vi "Get Channels limits.vi"(8 "error in (no error)":errorcluster, 9 "Power Supply In Use":T1, 10 "External Supply?":bool=TRUE, 11 "Channels":u16[](array[numeric])) -> (0 "error out":errorcluster, 3 "output cluster":T2)   [LabVIEW 2018, in "NI PXI-4110 Programmable Power Supply Custom Device.lvlib"]
uses:
  NI PXI-4110 Programmable Power Supply Custom Device.lvlib
  Power_Supply_In_Use.ctl
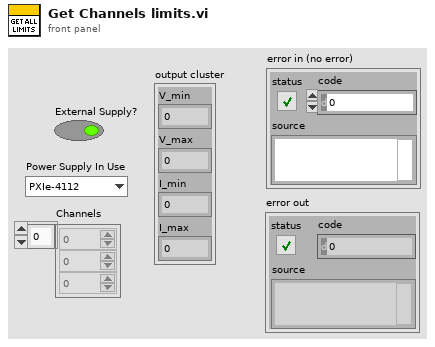
[diagram p1: front panel]
types:
  T1 = typedef "NI PXI-4110 Programmable Power Supply Custom Device.lvlib/Power_Supply_In_Use.ctl" = enum16{"PXIe-4112", "PXI-4110"}
  T2 = cluster{"V_min":dbl, "V_max":dbl, "I_min":dbl, "I_max":dbl}
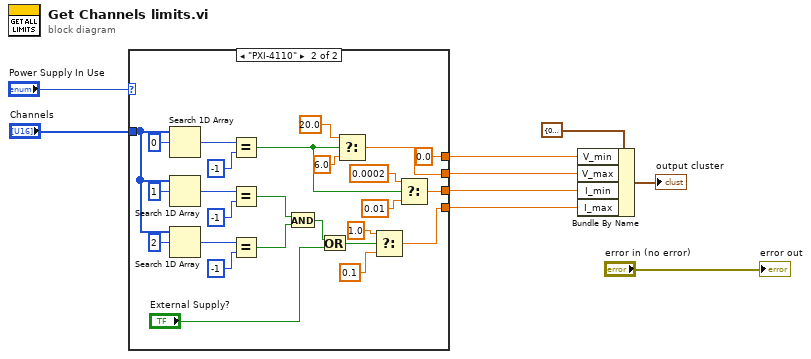
[diagram p0: block diagram]
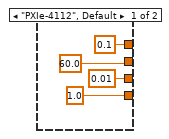
[diagram p2: hidden frame]
diagram:
  n1 = case shown="\"PXI-4110\"" "Power Supply In Use" {
    tunnel: [1.0 ("V_min") w21] -> w8
    tunnel: [0.01 ("V_min") w24] -> w7
    tunnel: [60.0 ("V_min") w26] -> w6
    tunnel: [0.1 ("V_min") 0.0 ("V_min")] -> w5
    tunnel: "Channels" -> [_ w30]
    frame "PXIe-4112", Default {
    }
    frame "PXI-4110" {
      n2 = Search 1D Array(1D array=w30, element=u16 0) -> (index of element=w38:i32)  [unwired: 1 in]
      n3 = Search 1D Array(1D array=w30, element=u16 1) -> (index of element=w35:i32)  [unwired: 1 in]
      n4 = Search 1D Array(1D array=w30, element=u16 2) -> (index of element=w32:i32)  [unwired: 1 in]
      n5 = Equal?(x=w38, y=-1) -> (x = y?=w25:bool)
      n6 = Equal?(x=w35, y=-1) -> (x = y?=w20:bool)
      n7 = Equal?(x=w32, y=-1) -> (x = y?=w19:bool)
      n8 = And(x=w20, y=w19) -> (x .and. y?=w18:bool)
      n9 = Or(x=w18, y="External Supply?") -> (x .or. y?=w16:bool)
      n10 = Select(t=20.0, s=w25, f=6.0) -> (s? t:f=w26:dbl)
      n11 = Select(t=1.0, s=w16, f=0.1) -> (s? t:f=w21:dbl)
      n12 = Select(t=0.0002, s=w25, f=0.01) -> (s? t:f=w24:dbl)
    }
  }
  n13 = Bundle By Name(cluster=T2 {"V_min"=0.0, "V_max"=0.0, "I_min"=0.0, "I_max"=0.0} ("output cluster"), "V_min"=w5, "V_max"=w6, "I_min"=w7, "I_max"=w8) -> (→"output cluster":T2)
  "error out" <- "error in (no error)"
